vi "DriveToDistance.vi"(8 "Error In":errorcluster, 10 "Setpoint":dbl) -> (0 "Error Out":errorcluster)   [LabVIEW 2016]
uses:
  <vilib>/Rock Robotics/WPI/Ultrasonic/WPI_SonarMB1010AnalogRefNum Registry Get.vi
  <vilib>/Rock Robotics/WPI/Ultrasonic/WPI_SonarMB1010AnalogGetRange.vi
  Robot Global Data.vi
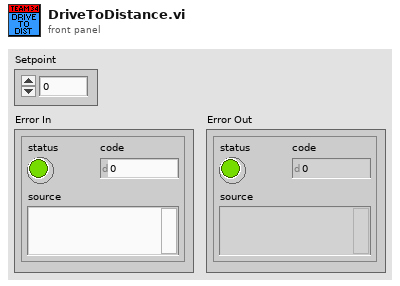
[diagram p1: front panel]
types:
  T1 = typedef "WPI_SonarMB1010AnalogDeviceRef.ctl" = cluster{"AIDeviceRef":T2, "Scaling factor (V/in)":dbl, "Average Bits":u8}
  T2 = typedef "WPI_AnalogChannelDevRef.ctl" = cluster{"DevStatus":errorcluster, "Analog Channel":T3}
  T3 = typedef "FPGA_AIChannel.ctl" = enum8{"AI 0", "AI 1", "AI 2", "AI 3", "AI MXP 0", "AI MXP 1", "AI MXP 2", "AI MXP 3", "Invalid"}
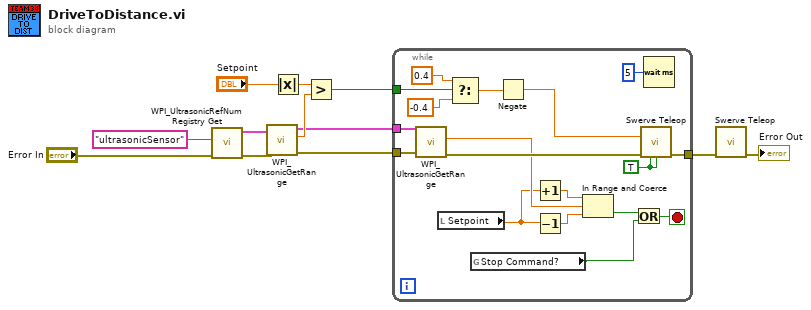
[diagram p0: block diagram]
diagram:
  n1 = call-poly <vilib>:"WPI_UltrasonicRefNum Registry Get.vi"("error in (no error)"="Error In", "refnum name"="ultrasonicSensor") -> ("error out"=w8:errorcluster, "SonarMB1010AnalogDevRef"=w6:T1)  [unwired: 8 in]
  n2 = call-poly <vilib>:"WPI_UltrasonicGetRange.vi"("error in"=w8, "SonarMB1010AnalogDevRef"=w6) -> ("error out"=w9:errorcluster, "Distance"=w10:dbl, "SonarMB1010AnalogDevRef"=w7:T1)  [unwired: 7 in]
  n3 = Absolute Value(x="Setpoint") -> (abs(x)=w11:dbl)
  n4 = Greater?(x=w11, y=w10) -> (0:w12:bool)
  n5 = while {
    tunnel: [w30] -> w5
    tunnel: w7 -> [w29]
    tunnel: w9 -> [w28]
    tunnel: w12 -> [w25]
    stop <- w16 stop-if-true
    w26 = TRUE ("Robot Centric?")
    n6 = call-poly <vilib>:"WPI_UltrasonicGetRange.vi"("error in"=w28, "SonarMB1010AnalogDevRef"=w29) -> ("error out"=w27:errorcluster, "Distance"=w21:dbl)  [unwired: 7 in, 1 out]
    n7 = local read "Setpoint"() -> (w17:dbl)
    n8 = Select(t=0.4, s=w25, f=-0.4) -> (s? t:f=w19:dbl)
    n9 = global read "Robot Global Data.vi" "Stop Command?"() -> (w14:bool)
    n10 = Negate(x=w19) -> (-x=w13:dbl)
    n11 = Increment(x=w17) -> (x+1=w23:dbl)
    n12 = Decrement(x=w17) -> (x-1=w22:dbl)
    n13 = In Range and Coerce(upper limit=w23, x=w21, lower limit=w22) -> (In Range?=w15:bool)  [unwired: 1 out]
    n14 = Or(x=w15, y=w14) -> (x .or. y?=w16:bool)
    n15 = call "Swerve Teleop.vi"("Y"=w13, "Error In"=w27, "Robot Centric?"=w26, "Autonomous?"=w26) -> ("Error Out"=w30:errorcluster)  [unwired: 7 in, 4 out]
    n16 = Wait (ms)(milliseconds to wait=u32 5) -> ()  [unwired: 1 out]
  }
  n17 = call "Swerve Teleop.vi"("Error In"=w5) -> ("Error Out"=→"Error Out":errorcluster)  [unwired: 10 in, 4 out]
